vi "GeneralGETwithSnapshot.vi"(6 "Dest Format":string(combo)="{6fddc324-4e03-4bfe-b185-3d77768dc90e}", 7 "HTTP_address":string, 10 "Value":T3, 11 "Refnum in":T2) -> (3 "headers":string)   [LabVIEW 2016]
uses:
  cgi_string.ctl
  <vilib>/httpClient/ClientHandle.ctl
  <vilib>/vision/Image Controls.llb/IMAQ Image.ctl
  <vilib>/httpClient/LabVIEWHTTPClient.lvlib
panel:
  out "Dest Format":string(combo)="{6fddc324-4e03-4bfe-b185-3d77768dc90e}"
  out "Image":T1(plugin-control)
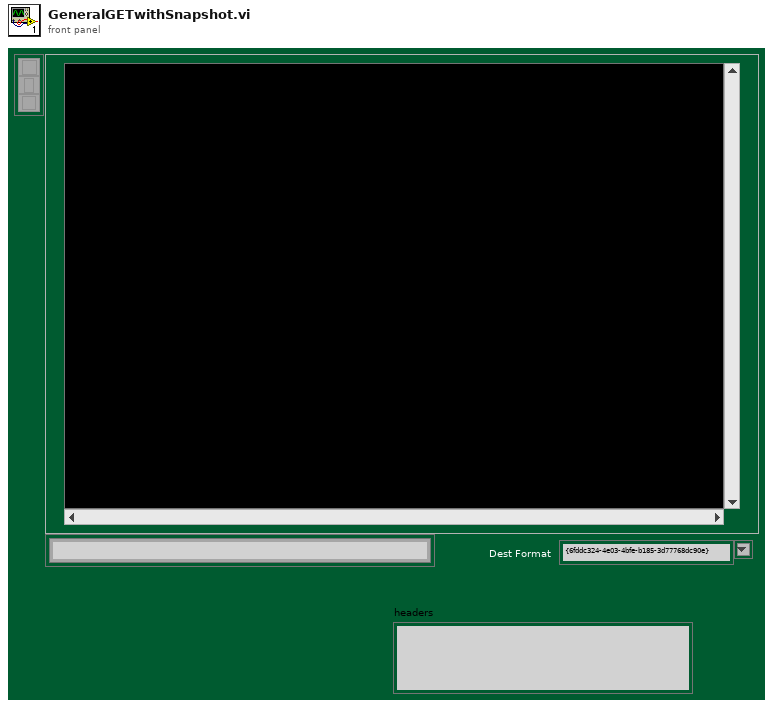
[diagram p1: front panel]
types:
  T1 = typedef "IMAQ Image.ctl" = refnum<image>
  T2 = typedef "LabVIEWHTTPClient.lvlib/ClientHandle.ctl" = refnum<k1>
  T3 = typedef "cgi_string.ctl" = string
  T4 = typedef "Image Type" = u32
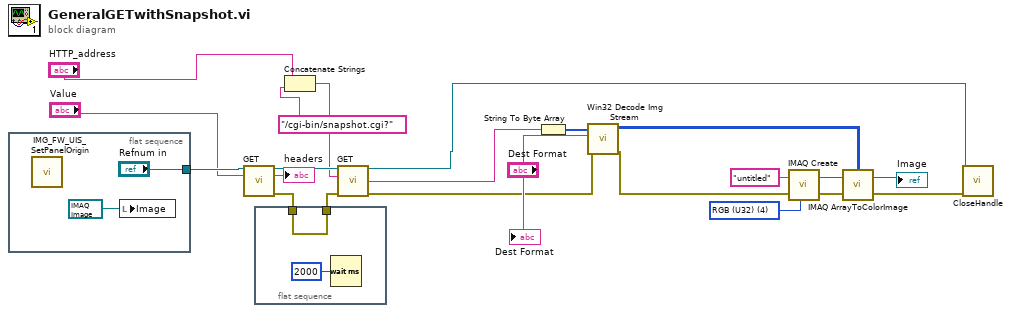
[diagram p0: block diagram]
diagram:
  w20 = T4 4 items=["Grayscale (U8)", "Grayscale (I16)", "Grayscale (SGL)", "Complex (CSG)", "RGB (U32)", "HSL (U32)", "RGB (U64)", "Grayscale (U16)"] ("Image Type")
  n1 = flat-sequence {
    tunnel: ["Refnum in"] -> w22
    frame #0 {
      n2 = call "IMG_FW_UIS_SetPanelOrigin.vi"() -> ()  [unwired: 11 in, 1 out]
      n3 = local write "Image"(T1 refnum ("New Image")) -> ()
    }
  }
  n4 = call <vilib>:"GET.vi"("client handle"=w22, "url"="Value") -> ("client handle out"=w10:T2, "headers"=→"headers":string, "error out"=w4:errorcluster)  [unwired: 10 in, 1 out]
  n5 = flat-sequence {
    tunnel: [w26] -> w3
    tunnel: w4 -> [w26]
    frame #0 {
      n6 = Wait (ms)(milliseconds to wait=u32 2000) -> ()  [unwired: 1 out]
    }
  }
  n7 = Concatenate Strings("HTTP_address", "/cgi-bin/snapshot.cgi?") -> (w5:string)
  n8 = call <vilib>:"GET.vi"("client handle"=w10, "url"=w5, "error in (no error)"=w3) -> ("client handle out"=w9:T2, "body"=w11:string, "error out"=w8:errorcluster)  [unwired: 9 in, 1 out]
  n9 = String To Byte Array(string=w11) -> (unsigned byte array=w18:u8[])
  n10 = call "Win32 Decode Img Stream.vi"("error in (no error)"=w8, "Dest Format"="Dest Format", "Image Data"=w18) -> ("error out"=w15:errorcluster, "Dest"=w17:u32[][])  [unwired: 4 in, 3 out]
  n11 = call "IMAQ Create"("Image Name"="untitled", "Image Type"=w20, "error in (no error)"=w15) -> ("New Image"=w21:T1, "error out"=w16:errorcluster)  [unwired: 2 in]
  n12 = call "IMAQ ArrayToColorImage"("Image Pixels (U32)"=w17, "Image"=w21, "error in (no error)"=w16) -> ("Image Out"=→"Image":T1, "error out"=w12:errorcluster)  [unwired: 2 in]
  n13 = call <vilib>:"CloseHandle.vi"("client handle"=w9, "error in (no error)"=w12) -> ()  [unwired: 13 in, 1 out]
  "Dest Format" <- "Dest Format"
